vi "날자의 참거짓 판별(SubVI).vi"() -> (1 "현재 날자":string, 2 "저장된 날자":string, 3 "불리언":bool)   [LabVIEW 2014]
uses:
  <vilib>/Utility/sysdir.llb/System Directory Type.ctl
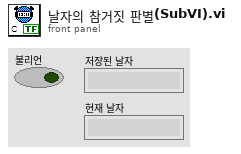
[diagram p1: front panel]
types:
  T1 = typedef "System Directory Type.ctl" = i32
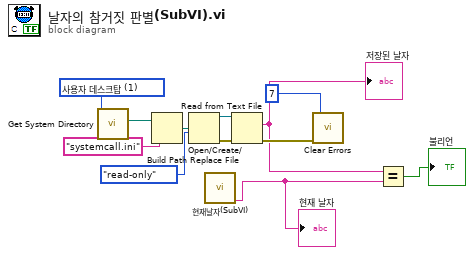
[diagram p0: block diagram]
diagram:
  w5 = T1 1 items=["사용자 홈"=0, "사용자 데스크탑"=1, "사용자 문서"=2, "사용자 어플리케이션 데이터"=3, "사용자 환경"=4, "사용자 임시"=5, "퍼블릭 문서"=6, "퍼블릭 어플리케이션 데이터"=7, "퍼블릭 환경"=8, "퍼블릭 캐시"=13, "시스템 코어 라이브러리"=9, "시스템 설치된 라이브러리"=10, "어플리케이션 파일"=11, "부팅 볼륨 루트"=12] ("system directory type")
  n1 = call <vilib>:"Get System Directory.vi"("system directory type"=w5) -> ("system directory"=w6:path)  [unwired: 10 in]
  n2 = Build Path(base path=w6, name or relative path="systemcall.ini" ("이름 또는 상대 경로")) -> (appended path=w8:path)
  n3 = Open/Create/Replace File(file path (use dialog)=w8, access (0:read/write)=enum16{"read/write", "read-only", "write-only"}."read-only" ("접근(0:읽기/쓰기)")) -> (refnum out=w10:refnum<file>, error out=w11:errorcluster)  [unwired: 4 in, 1 out]
  n4 = call "현재날자(SubVI).vi"() -> ("월,일 을 문자열로"=w1:string)  [unwired: 5 in, 6 out]
  "현재 날자" <- w1
  n5 = Read from Text File(file (use dialog)=w10, error in=w11) -> (text=w2:string, error out=w3:errorcluster)  [unwired: 2 in, 2 out]
  "저장된 날자" <- w2
  n6 = call <vilib>:"Clear Errors.vi"("error in (no error)"=w3, "specific error code to clear (0: all)"=7) -> ()  [unwired: 4 in, 2 out]
  n7 = Equal?(x=w2, y=w1) -> (x = y?=→"불리언":bool)
